vi "Read Power Impl.vi"(8 "error in (no error)":errorcluster, 11 "Newport Power Meter in":refnum<class "Newport Power Meter.lvclass">) -> (0 "error out":errorcluster, 2 "Raw Device Reading (W)":dbl=-1.0 caption="Power", 3 "Newport Power Meter out":refnum<class "Newport Power Meter.lvclass">)   [LabVIEW 2023, in "Newport Power Meter.lvlib" / "Newport Power Meter.lvclass"]
uses:
  Newport Power Meter.lvclass
  Newport Power Meter.lvclass/Newport Power Meter.ctl
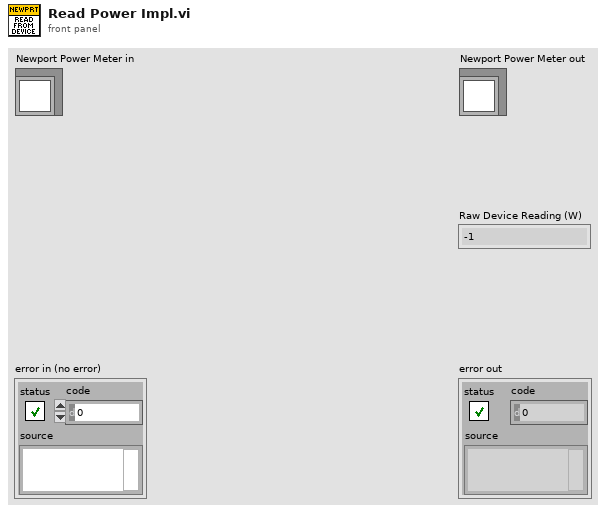
[diagram p1: front panel]
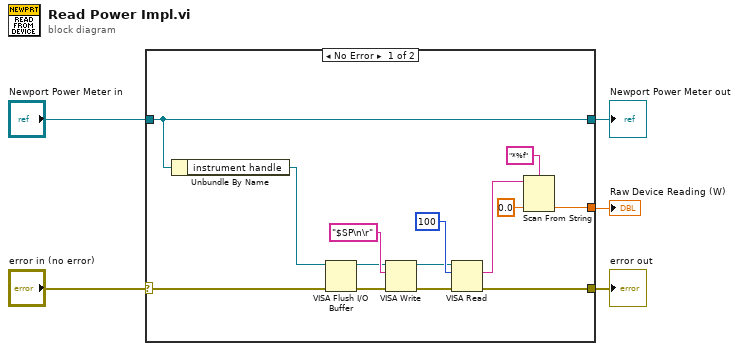
[diagram p0: block diagram]
diagram:
  n1 = case shown="No Error" "error in (no error)" {
    selector: "error in (no error)" -> [w11 w20]
    tunnel: "Newport Power Meter in" -> [w9 w21]
    tunnel: [w9 w21] -> w4
    tunnel: [w6 w20] -> w2
    tunnel: [w7 _] -> w1
    frame No Error {
      n2 = Unbundle By Name(w9) -> ("instrument handle"=w8:refnum<visa-resource-name>)
      n3 = VISA Flush I/O Buffer(VISA resource name=w8, error in (no error)=w11) -> (VISA resource name out=w17:refnum<visa-resource-name>, error out=w18:errorcluster)  [unwired: 1 in]
      n4 = VISA Write(VISA resource name=w17, write buffer="$SP\n\r", error in (no error)=w18) -> (VISA resource name out=w15:refnum<visa-resource-name>, error out=w14:errorcluster)  [unwired: 1 out]
      n5 = VISA Read(VISA resource name=w15, byte count=u32 100, error in (no error)=w14) -> (read buffer=w13:string, error out=w6:errorcluster)  [unwired: 2 out]
      n6 = Scan From String(format string="*%f", input string=w13, default 1=0.0 ("default value 1")) -> (output 1=w7:dbl)  [unwired: 2 in, 3 out]
    }
    frame Error {
    }
  }
  "error out" <- w2
  "Newport Power Meter out" <- w4
  "Raw Device Reading (W)" <- w1
